vi "qn_get direction.vi"(7 "reset":bool, 8 "error in (no error)":errorcluster, 10 "gradient":dbl[](array[numeric]), 11 "X":dbl[](array[numeric])) -> (0 "error out":errorcluster, 3 "direction":dbl[](array[numeric]))   [LabVIEW 2024, in "NI_Gmath.lvlib"]
uses:
  NI_Gmath.lvlib
  A x Vector.vi
  NI_AALBase.lvlib
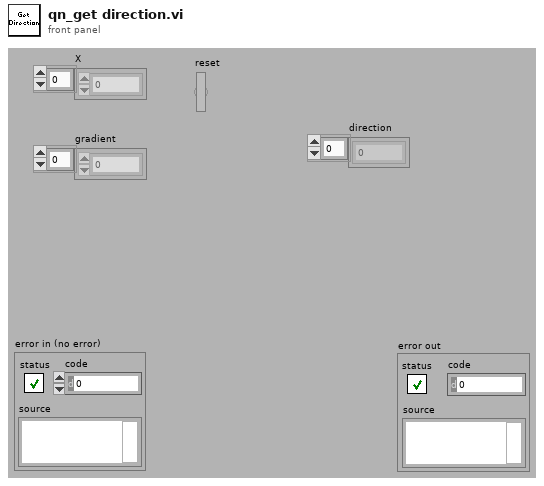
[diagram p1: front panel]
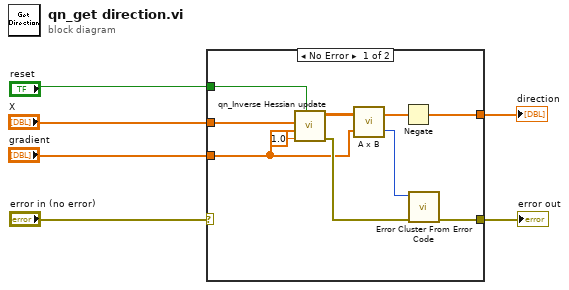
[diagram p0: block diagram]
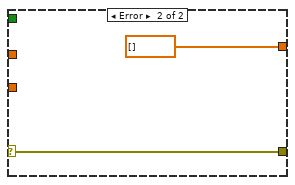
[diagram p2: hidden frame]
diagram:
  n1 = case shown="No Error" "error in (no error)" {
    selector: "error in (no error)" -> [_ w18]
    tunnel: [w15 dbl[] []] -> w6
    tunnel: [w8 w18] -> w5
    tunnel: "X" -> [w11 _]
    tunnel: "gradient" -> [w10 _]
    tunnel: "reset" -> [w7 _]
    frame No Error {
      n2 = call "qn_Inverse Hessian update.vi"("reset"=w7, "zeta"=1.0, "gradient"=w10, "X"=w11) -> ("error out"=w16:errorcluster, "Dk+1"=w13:dbl[][])  [unwired: 6 in]
      n3 = call-poly "A x B.vi"("Vector"=w10, "A"=w13) -> ("error"=w9:i32, "A x Vector"=w14:dbl[])
      n4 = Negate(x=w14) -> (-x=w15:dbl[])
      n5 = call "Error Cluster From Error Code.vi"("error in (no error)"=w16, "error code (0)"=w9) -> ("error out"=w8:errorcluster)  [unwired: 7 in]
    }
    frame Error {
    }
  }
  "direction" <- w6
  "error out" <- w5
